vi "Sound Signal.vi"(8 "error in (no error)":errorcluster, 11 "Bicycle in":refnum<class "Bicycle.lvclass">) -> (0 "error out":errorcluster, 3 "Bicycle out":refnum<class "Bicycle.lvclass">)   [LabVIEW 2019, in "Bicycle.lvclass"]
uses:
  Bicycle.lvclass
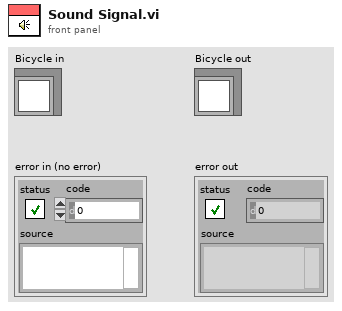
[diagram p1: front panel]
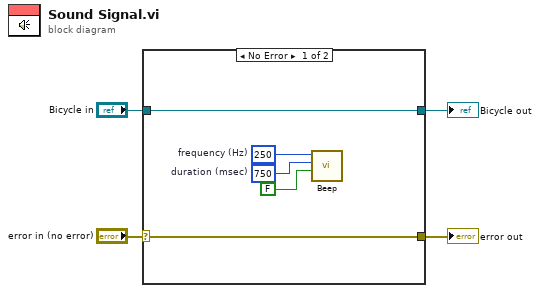
[diagram p0: block diagram]
diagram:
  n1 = case shown="No Error" "error in (no error)" {
    selector: "error in (no error)" -> [w8 w10]
    tunnel: "Bicycle in" -> [w9 w11]
    tunnel: [w9 w11] -> w2
    tunnel: [w8 w10] -> w1
    frame No Error {
      w5 = u32 750  # duration (msec)
      w6 = u32 250  # frequency (Hz)
      n2 = call <vilib>:"Beep.vi"("use system alert? (T)"=FALSE, "duration (msec)"=w5, "frequency (Hz)"=w6) -> ()  [unwired: 9 in]
    }
    frame Error {
    }
  }
  "error out" <- w1
  "Bicycle out" <- w2
